vi "Read Data.vi"(7 "SlaveID":u8=1, 8 "error in (no error)":errorcluster, 9 "# samples to read":u16, 11 ".NET Refnum in":refnum<k24>) -> (0 "error out":errorcluster, 1 "# samples in buffer":u16, 2 "Vib":u16[](array[numeric]), 3 "reference out":refnum<k24>)   [LabVIEW 2017]
uses:
  dll/Modbus.dll
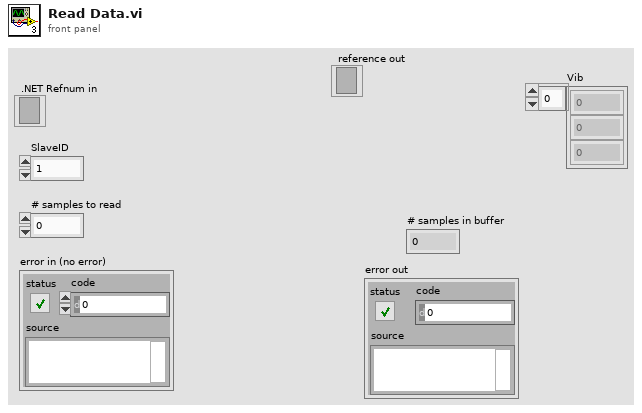
[diagram p1: front panel]
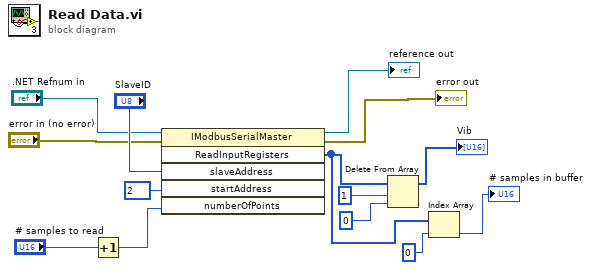
[diagram p0: block diagram]
diagram:
  n1 = Increment(x="# samples to read") -> (x+1=w2:u16)
  n2 = invoke class="IModbusSerialMaster" method="ReadInputRegisters"(reference=".NET Refnum in", error in="error in (no error)", "slaveAddress"="SlaveID", "startAddress"=u16 2, "numberOfPoints"=w2) -> (reference out=→"reference out":refnum<k24>, error out=→"error out":errorcluster, "ReadInputRegisters"=w3:u16[])  [unwired: 1 in, 3 out]
  n3 = Delete From Array(array=w3, length=1, index=0) -> (array with subset deleted=→"Vib":u16[])  [unwired: 1 out]
  n4 = Index Array(array=w3, index=0) -> (element=→"# samples in buffer":u16)
